vi "Day 05 (Part One).vi"() -> ()   [LabVIEW 2021]
panel:
  out "result":u32
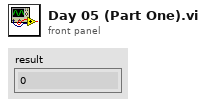
[diagram p1: front panel]
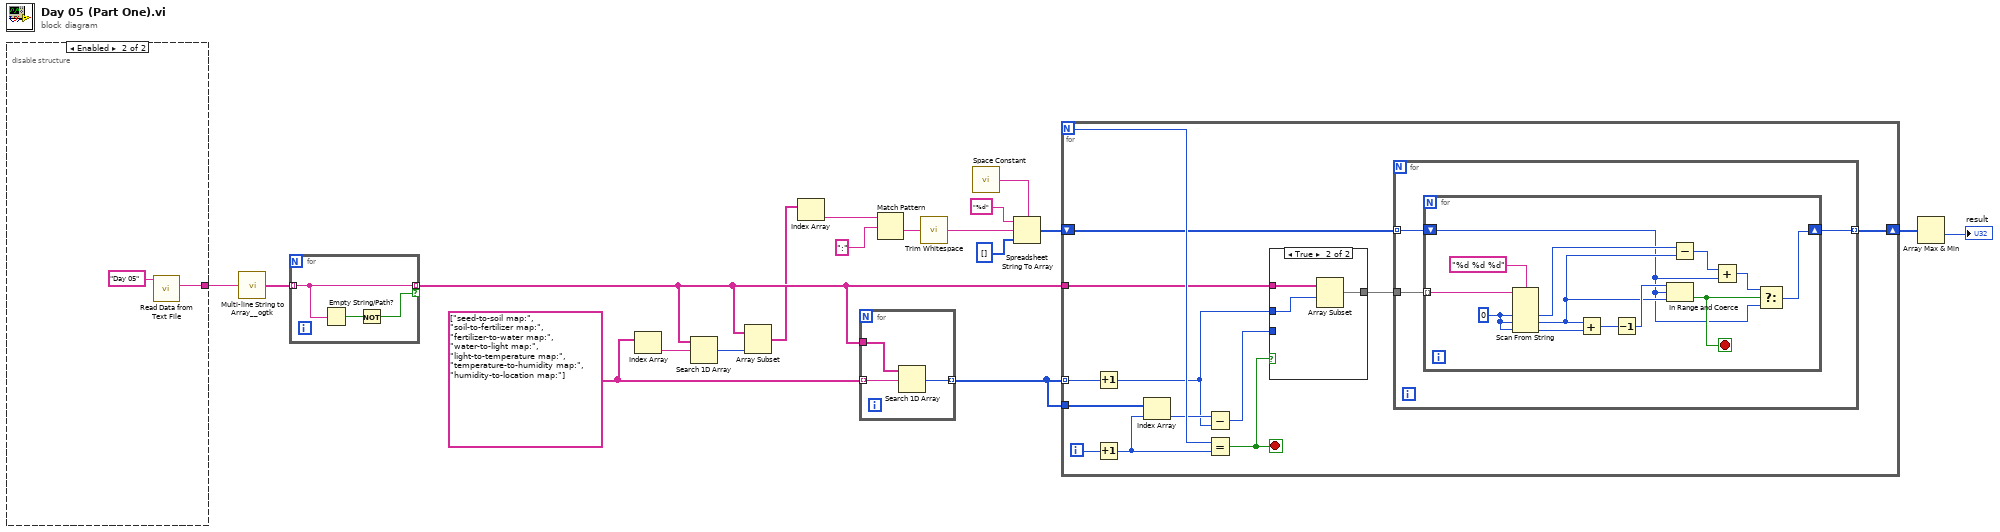
[diagram p0: block diagram]
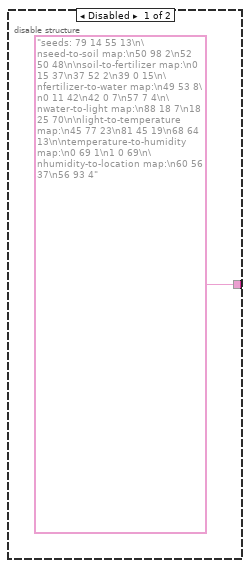
[diagram p2: hidden frame]
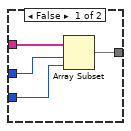
[diagram p3: hidden frame]
diagram:
  w15 = string[] ["seed-to-soil map:", "soil-to-fertilizer map:", "fertilizer-to-water map:", "water-to-light map:", "light-to-temperature map:", "temperature-to-humidity map:", "humidity-to-location map:"]
  n1 = disable-structure shown="Enabled" {
    disable-tunnel: ["seeds: 79 14 55 13\n\nseed-to-soil map:\n50 98 2\n52 50 48\n\nsoil-to-fertilizer map:\n0 15 37\n37 52 2\n39 0 15\n\nfertilizer-to-water map:\n49 53 8\n0 11 42\n42 0 7\n57 7 4\n\nwater-to-light map:\n88 18 7\n18 25 70\n\nlight-to-temperature map:\n45 77 23\n81 45 19\n68 64 13\n\ntemperature-to-humidity map:\n0 69 1\n1 0 69\n\nhumidity-to-location map:\n60 56 37\n56 93 4" w21] -> w18
    frame Disabled {
    }
    frame Enabled {
      n2 = call "Read Data from Text File.vi"("Subfolder"="Day 05") -> ("data"=w21:string)  [unwired: 10 in]
    }
  }
  n3 = call <userlib>:"Multi-line String to Array__ogtk.vi"("string"=w18) -> ("lines"=w13:string[])
  n4 = for {
    tunnel: w13 -> [w23] mode=indexing
    tunnel: [w23] -> w12 mode=indexing if=w22
    n5 = Empty String/Path?(string/path=w23) -> (empty?=w24:bool)
    n6 = Not(x=w24) -> (.not. x?=w22:bool)
  }
  n7 = Index Array(array=w15) -> (element=w17:string)  [unwired: 1 in]
  n8 = Search 1D Array(1D array=w12, element=w17) -> (index of element=w16:i32)  [unwired: 1 in]
  n9 = Array Subset(array=w12, length=w16) -> (w11:string[])  [unwired: 1 in]
  n10 = Index Array(array=w11) -> (element=w10:string)  [unwired: 1 in]
  n11 = for {
    tunnel: w15 -> [w27] mode=indexing
    tunnel: [w26] -> w14 mode=indexing
    tunnel: w12 -> [w25]
    n12 = Search 1D Array(1D array=w25, element=w27) -> (index of element=w26:i32)  [unwired: 1 in]
  }
  n13 = Match Pattern(string=w10, regular expression=":") -> (after substring=w8:string)  [unwired: 1 in, 3 out]
  n14 = call <vilib>:"Trim Whitespace.vi"("string"=w8) -> ("trimmed string"=w7:string)  [unwired: 1 in]
  n15 = call <vilib>:"Space Constant.vi"() -> ("String"=w5:string)
  n16 = Spreadsheet String To Array(delimiter (Tab)=w5, format string="%d", spreadsheet string=w7, array type (2D Dbl)=u32[] []) -> (array=w3:u32[])
  n17 = for {
    N -> [w37]
    tunnel: w14 -> [w33] mode=indexing
    tunnel: w14 -> [w39]
    tunnel: w12 -> [w36]
    shift-right: [w28] -> w2
    shift-left: w3 -> [w30]
    i -> [w40]
    stop <- w32 stop-if-true
    n18 = Increment(x=w33) -> (x+1=w31:i32)
    n19 = Increment(x=w40) -> (x+1=w38:i32)
    n20 = Index Array(array=w39, index=w38) -> (element=w35:i32)
    n21 = Subtract(x=w35, y=w31) -> (x-y=w34:i32)
    n22 = Equal?(x=w37, y=w38) -> (x = y?=w32:bool)
    n23 = case shown="True" w32 {
      tunnel: w36 -> [w60 w63]
      tunnel: w34 -> [w59 _]
      tunnel: w31 -> [w58 w61]
      tunnel: [w57 w62] -> w29
      frame False {
        n24 = Array Subset(array=w60, index=w58, length=w59) -> (w57:string[])
      }
      frame True {
        n25 = Array Subset(array=w63, index=w61) -> (w62:string[])  [unwired: 1 in]
      }
    }
    n26 = for {
      tunnel: w29 -> [w43]
      tunnel: w30 -> [w42] mode=indexing
      tunnel: [w41] -> w28 mode=indexing
      n27 = for {
        tunnel: w43 -> [w56] mode=indexing
        shift-right: [w49] -> w41
        shift-left: w42 -> [w44]
        stop <- w51 stop-if-true
        w46 = u32 0 ("default value 1")
        n28 = Scan From String(format string="%d %d %d", input string=w56, default 1=w46, default 2=w46, default 3=w46) -> (output 1=w45:u32, output 2=w47:u32, output 3=w54:u32)  [unwired: 2 in, 3 out]
        n29 = Add(x=w47, y=w54) -> (x+y=w53:u32)
        n30 = Decrement(x=w53) -> (x-1=w48:u32)
        n31 = In Range and Coerce(upper limit=w48, x=w44, lower limit=w47) -> (In Range?=w51:bool)  [unwired: 1 out]
        n32 = Subtract(x=w45, y=w47) -> (x-y=w52:u32)
        n33 = Add(x=w52, y=w44) -> (x+y=w50:u32)
        n34 = Select(t=w50, s=w51, f=w44) -> (s? t:f=w49:u32)
      }
    }
  }
  n35 = Array Max & Min(array=w2) -> (min value=→"result":u32)  [unwired: 3 out]
